vi "DriveExecuteTestFeedFowardKa.vi"(8 "error in (no error)":errorcluster) -> (0 "error out":errorcluster)   [LabVIEW 2023]
doc: "Execute and test/tune feed foward for Drive\n\nClosed control loop for drive\n\ninput: \n error in (cluster)\n\noutput:\n error out (cluster)"
uses:
  <vilib>/Rock Robotics/WPI/ThirdParty/Phoenix-LabVIEW/Motor Controller/Controls/CTRE_Phoenix_MotorControl_ControlMode.ctl
  DriveGlobal.vi
  <vilib>/Rock Robotics/WPI/ThirdParty/JAS_Junk/TrajLib/Trajectory_Library.lvlib
  <vilib>/Rock Robotics/Network Tables/NT Write Number.vi
  <vilib>/Rock Robotics/Network Tables/NT Write Boolean.vi
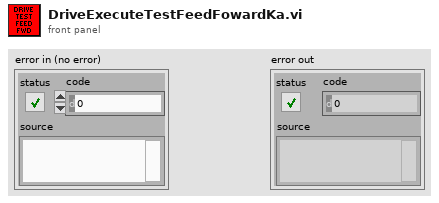
[diagram p1: front panel]
types:
  T1 = typedef "CTRE_Phoenix_MotorControl_ControlMode.ctl" = u16
  T2 = typedef "ADIS16470 Device Reference.ctl" = cluster{"DevStatus":errorcluster, "Hardware Config":T3, "Calibration Complete":refnum<notifier>, "Status Reference":refnum<data-value>, "Data Reference":refnum<data-value>, "Sychronous Process VI":T7, "Cmd FIFO":refnum<k33>, "Source":T8, "Data FIFO":refnum<k33>, "Calibration Time (ms)":u32, "Data Reference":refnum<data-value>}
  T3 = typedef "ADIS16470 Hardware Configuration.ctl" = cluster{"SPI Clock Rate (Hz)":dbl, "IMU SPI Mode (3)":T4, "IMU Reset Pin":T5, "IMU SPI Bus":T6, "IMU Data Ready Pin":T5, "Stall Config":cluster{"Pow2BytesPerRead":u8, "StallTicks":u16, "CsToSclkTicks":u8}}
  T4 = typedef "WPI_SPIMode.ctl" = enum16{"Mode 0 (Clk Idle Low,Sample on Leading)", "Mode 1 (Clk Idle Low,Sample on Trailing)", "Mode 2 (Clk Idle High,Sample on Leading)", "Mode 3 (Clk Idle High,Sample on Trailing)"}
  T5 = typedef "FPGA_DIOChannel.ctl" = enum8{"DIO 0", "DIO 1", "DIO 2", "DIO 3", "DIO 4", "DIO 5", "DIO 6", "DIO 7", "DIO 8", "DIO 9", "DIO MXP 0", "DIO MXP 1", "DIO MXP 2", "DIO MXP 3", "DIO MXP 4", "DIO MXP 5", "DIO MXP 6", "DIO MXP 7", "DIO MXP 8", "DIO MXP 9", "DIO MXP 10", "DIO MXP 11", "DIO MXP 12", "DIO MXP 13", "DIO MXP 14", "DIO MXP 15", "SPI Port CS1", "SPI Port CS2", "SPI Port CS3", "SPI Port MISO", "SPI Port MOSI", "Invalid"}
  T6 = typedef "spi_bus.ctl" = enum16{"SPI On-Board, CS0", "SPI On-Board, CS1", "SPI On-Board, CS2", "SPI On-Board, CS3", "SPI MXP", "Invalid"}
  T7 = typedef "ADIS16470 Process.ctl" = refnum<vi>
  T8 = typedef "FPGA_CounterEncoderSourceConvertionLVSourceType.ctl" = cluster{"DevStatus":errorcluster, "AnalogTriggerMode?":bool, "DigitalMode":cluster{"DIO Channel":T9}, "AnalogTriggerMode":cluster{"AnalogTriggerIndex":T10, "OutputType":T11}}
  T9 = typedef "FPGA_DIODigitalSourceChannel.ctl" = enum8{"DIO 0", "DIO 1", "DIO 2", "DIO 3", "DIO 4", "DIO 5", "DIO 6", "DIO 7", "DIO 8", "DIO 9", "DIO MXP 0", "DIO MXP 1", "DIO MXP 2", "DIO MXP 3", "DIO MXP 4", "DIO MXP 5", "DIO MXP 6", "DIO MXP 7", "DIO MXP 8", "DIO MXP 9", "DIO MXP 10", "DIO MXP 11", "DIO MXP 12", "DIO MXP 13", "DIO MXP 14", "DIO MXP 15", "SPI Port CS1", "SPI Port CS2", "SPI Port CS3", "SPI Port MISO", "SPI Port MOSI", "Disabled"}
  T10 = typedef "FPGA_AnalogTriggerIndex.ctl" = enum8{"Trig 0", "Trig 1", "Trig 2", "Trig 3", "Trig 4", "Trig 5", "Trig 6", "Trig 7", "Invalid"}
  T11 = typedef "FPGA_AnalogTriggerOutType.ctl" = enum16{"InWindow", "TriggerState", "Rising", "Falling"}
  T12 = typedef "ADIS16470 Data.ctl" = cluster{"XAngle":dbl, "YAngle":dbl, "ZAngle":dbl}
  T13 = typedef "Trajectory_Library.lvlib/SIMPLE_MOTOR_FF_KA_TUNE_PARAMS.ctl" = cluster{"Max SP":dbl, "Min Eval SP":dbl, "Max Eval SP":dbl, "Ramp Rate":dbl}
  T14 = typedef "Trajectory_Library.lvlib/SIMPLE_MOTOR_FF.ctl" = cluster{"Ks":dbl, "Kv":dbl, "Ka":dbl, "KnInv":dbl}
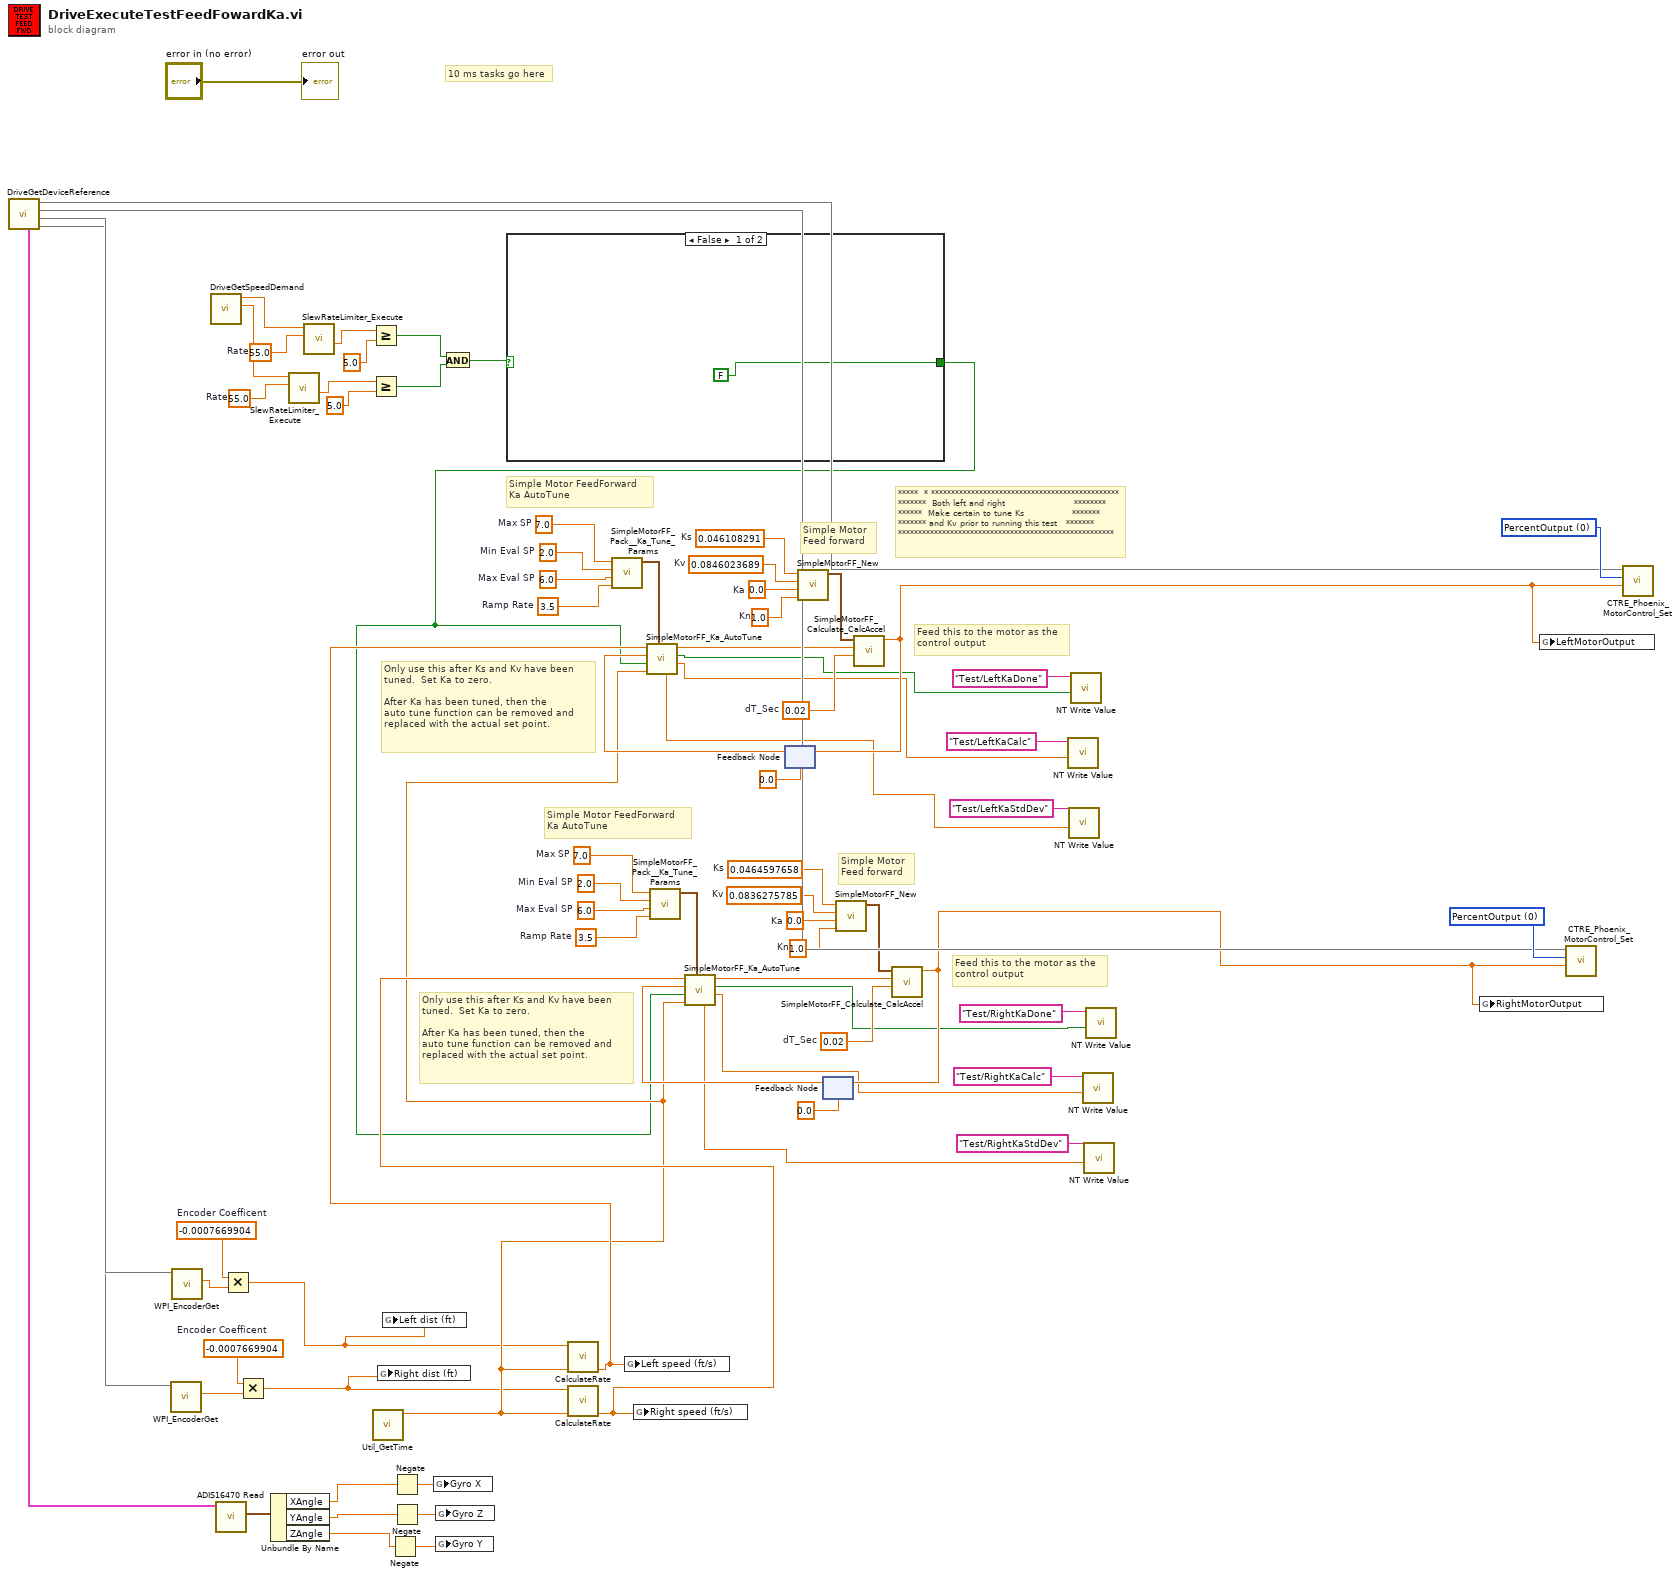
[diagram p0: block diagram]
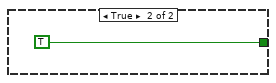
[diagram p2: hidden frame]
diagram:
  w7 = -0.0007669904  # Encoder Coefficent
  w8 = -0.0007669904  # Encoder Coefficent
  w36 = 1.0  # Kn
  w35 = 0.02  # dT_Sec
  w33 = 0.0464597658  # Ks
  w32 = 0.0836275785  # Kv
  w31 = 0.0  # Ka
  w30 = 7.0  # Max SP
  w29 = 2.0  # Min Eval SP
  w28 = 6.0  # Max Eval SP
  w27 = 3.5  # Ramp Rate
  w51 = 1.0  # Kn
  w50 = 0.02  # dT_Sec
  w48 = 0.046108291  # Ks
  w47 = 0.0846023689  # Kv
  w46 = 0.0  # Ka
  w45 = 7.0  # Max SP
  w44 = 2.0  # Min Eval SP
  w43 = 6.0  # Max Eval SP
  w42 = 3.5  # Ramp Rate
  w69 = 55.0  # Rate
  w71 = 55.0  # Rate
  w77 = T1 0 items=["PercentOutput"=0, "Position"=1, "Velocity"=2, "Current"=3, "Follower"=5, "MotionProfile"=6, "MotionMagic"=7, "MotionProfileArc"=10, "Disabled"=15] ("Control Mode")
  w78 = T1 0 items=["PercentOutput"=0, "Position"=1, "Velocity"=2, "Current"=3, "Follower"=5, "MotionProfile"=6, "MotionMagic"=7, "MotionProfileArc"=10, "Disabled"=15] ("Control Mode")
  # "*****  * ***********************************************\n*******  Both left and right                       ********  \n******  Make certain to tune Ks                *******\n******* and Kv prior to running this test   *******\n******************************************************"
  # "Only use this after Ks and Kv have been\ntuned.  Set Ka to zero.\n\nAfter Ka has been tuned, then the \nauto tune function can be removed and\nreplaced with the actual set point."
  # "Feed this to the motor as the\ncontrol output"
  # "Simple Motor\nFeed forward"
  # "Simple Motor FeedForward\nKa AutoTune"
  # "Only use this after Ks and Kv have been\ntuned.  Set Ka to zero.\n\nAfter Ka has been tuned, then the \nauto tune function can be removed and\nreplaced with the actual set point."
  # "Feed this to the motor as the\ncontrol output"
  # "Simple Motor\nFeed forward"
  # "Simple Motor FeedForward\nKa AutoTune"
  # "10 ms tasks go here"
  n1 = call "DriveGetDeviceReference.vi"() -> (0:w1, 1:w2, 2:w72, 3:w73, "Gryo"=w74:T2)  [unwired: 7 in]
  n2 = call <vilib>:"WPI_EncoderGet.vi"("EncoderDevRef"=w1) -> ("Distance"=w5:dbl)  [unwired: 5 in, 5 out]
  n3 = call <vilib>:"WPI_EncoderGet.vi"("EncoderDevRef"=w2) -> ("Distance"=w6:dbl)  [unwired: 5 in, 5 out]
  n4 = call "DriveGetSpeedDemand.vi"() -> ("vY"=w68:dbl, "vX"=w70:dbl)  [unwired: 8 in, 2 out]
  n5 = call <vilib>:"ADIS16470 Read.vi"("ADIS16470DevRef"=w74) -> ("ADIS16470 Value"=w75:T12)  [unwired: 7 in, 3 out]
  n6 = Multiply(x=w8, y=w6) -> (x*y=w3:dbl)
  n7 = Multiply(x=w7, y=w5) -> (x*y=w4:dbl)
  n8 = Unbundle By Name(w75) -> ("XAngle"=w62:dbl, "YAngle"=w64:dbl, "ZAngle"=w63:dbl)
  n9 = call <vilib>:"SlewRateLimiter_Execute.vi"("PositiveRate"=w69, "Input"=w68) -> ("Output"=w55:dbl)  [unwired: 8 in, 1 out]
  n10 = call <vilib>:"SlewRateLimiter_Execute.vi"("PositiveRate"=w71, "Input"=w70) -> ("Output"=w56:dbl)  [unwired: 8 in, 1 out]
  n11 = Greater Or Equal?(x=w56, y=5.0) -> (x >= y?=w59:bool)
  n12 = Greater Or Equal?(x=w55, y=5.0) -> (x >= y?=w58:bool)
  n13 = call <vilib>:"Util_GetTime.vi"() -> ("FPGA_Time_Seconds"=w10:dbl)  [unwired: 9 in, 2 out]
  n14 = global write "DriveGlobal.vi" "Right dist (ft)"(w4) -> ()
  n15 = global write "DriveGlobal.vi" "Left dist (ft)"(w3) -> ()
  n16 = Negate(x=w63) -> (-x=w66:dbl)
  n17 = Negate(x=w62) -> (-x=w67:dbl)
  n18 = Negate(x=w64) -> (-x=w65:dbl)
  n19 = global write "DriveGlobal.vi" "Gyro X"(w67) -> ()
  n20 = global write "DriveGlobal.vi" "Gyro Z"(w65) -> ()
  n21 = global write "DriveGlobal.vi" "Gyro Y"(w66) -> ()
  n22 = And(x=w59, y=w58) -> (x .and. y?=w57:bool)
  n23 = case shown="False" w57 {
    tunnel: [FALSE TRUE] -> w9
    frame False {
    }
    frame True {
    }
  }
  n24 = call "CalculateRate.vi"("Time (s)"=w10, "Distance (units)"=w3) -> ("Rate (units/s)"=w40:dbl)  [unwired: 9 in]
  n25 = call "CalculateRate.vi"("Time (s)"=w10, "Distance (units)"=w4) -> ("Rate (units/s)"=w25:dbl)  [unwired: 9 in]
  n26 = call <vilib>:"SimpleMotorFF_Pack__Ka_Tune_Params.vi"("Ramp Rate"=w42, "Max Eval SP"=w43, "Min Eval SP"=w44, "Max SP"=w45) -> ("Packed Params"=w41:T13)  [unwired: 7 in]
  n27 = global write "DriveGlobal.vi" "Left speed (ft/s)"(w40) -> ()
  n28 = global write "DriveGlobal.vi" "Right speed (ft/s)"(w25) -> ()
  n29 = call <vilib>:"SimpleMotorFF_Pack__Ka_Tune_Params.vi"("Ramp Rate"=w27, "Max Eval SP"=w28, "Min Eval SP"=w29, "Max SP"=w30) -> ("Packed Params"=w26:T13)  [unwired: 7 in]
  n30 = feedback #1(0.0 ("FeedForward")) -> (w53:dbl)
  n31 = call <vilib>:"SimpleMotorFF_Ka_AutoTune.vi"("SimpleMotorFeedforward_KaTune_Pack"=w41, "PassThroughTime"=w10, "Run Test"=w9, "CO Control Output"=w53, "PV ProcessVariable"=w40) -> ("Ka Calc"=w21:dbl, "Test Complete"=w22:bool, "SP Setpoint"=w52:dbl, "Ka StdDev"=w17:dbl)  [unwired: 3 out]
  n32 = call <vilib>:"SimpleMotorFF_New.vi"("Kn"=w51, "Ka"=w46, "Kv"=w47, "Ks"=w48) -> ("SIMPLE_MOTOR_FF"=w49:T14)  [unwired: 7 in]
  n33 = feedback #2(0.0 ("FeedForward")) -> (w38:dbl)
  n34 = call <vilib>:"SimpleMotorFF_Ka_AutoTune.vi"("SimpleMotorFeedforward_KaTune_Pack"=w26, "PassThroughTime"=w10, "Run Test"=w9, "CO Control Output"=w38, "PV ProcessVariable"=w25) -> ("Ka Calc"=w12:dbl, "Test Complete"=w13:bool, "SP Setpoint"=w37:dbl, "Ka StdDev"=w11:dbl)  [unwired: 3 out]
  n35 = call <vilib>:"SimpleMotorFF_New.vi"("Kn"=w36, "Ka"=w31, "Kv"=w32, "Ks"=w33) -> ("SIMPLE_MOTOR_FF"=w34:T14)  [unwired: 7 in]
  n36 = call <vilib>:"SimpleMotorFF_Calculate_CalcAccel.vi"("dT_Sec"=w50, "VelSp"=w52, "SIMPLE_MOTOR_FF"=w49) -> ("FeedForward"=w24:dbl)  [unwired: 8 in]
  n37 = feedback-in #1(w24) -> ()
  n38 = call <vilib>:"SimpleMotorFF_Calculate_CalcAccel.vi"("dT_Sec"=w35, "VelSp"=w37, "SIMPLE_MOTOR_FF"=w34) -> ("FeedForward"=w23:dbl)  [unwired: 8 in]
  n39 = feedback-in #2(w23) -> ()
  n40 = call-poly <vilib>:"NT Write Value.vi"("value"=w21, "name"="Test/LeftKaCalc") -> ()  [unwired: 9 in, 1 out]
  n41 = call-poly <vilib>:"NT Write Value.vi"("value"=w17, "name"="Test/LeftKaStdDev") -> ()  [unwired: 9 in, 1 out]
  n42 = call-poly <vilib>:"NT Write Value.vi"("value"=w22, "name"="Test/LeftKaDone") -> ()  [unwired: 9 in, 1 out]
  n43 = call-poly <vilib>:"NT Write Value.vi"("value"=w12, "name"="Test/RightKaCalc") -> ()  [unwired: 9 in, 1 out]
  n44 = call-poly <vilib>:"NT Write Value.vi"("value"=w11, "name"="Test/RightKaStdDev") -> ()  [unwired: 9 in, 1 out]
  n45 = call-poly <vilib>:"NT Write Value.vi"("value"=w13, "name"="Test/RightKaDone") -> ()  [unwired: 9 in, 1 out]
  n46 = global write "DriveGlobal.vi" "RightMotorOutput"(w23) -> ()
  n47 = global write "DriveGlobal.vi" "LeftMotorOutput"(w24) -> ()
  n48 = call <vilib>:"CTRE_Phoenix_MotorControl_Set.vi"("Output"=w23, "Control Mode"=w77, "PhoenixMotorControlDevRef"=w72) -> ()  [unwired: 7 in, 2 out]
  n49 = call <vilib>:"CTRE_Phoenix_MotorControl_Set.vi"("Output"=w24, "Control Mode"=w78, "PhoenixMotorControlDevRef"=w73) -> ()  [unwired: 7 in, 2 out]
  "error out" <- "error in (no error)"
